vi "ChangeExecTimeCmdCluster.vi"(9 "ExecTime":string, 11 "CmdClusterIN":T2) -> (3 "CmdClusterOUT":T1)   [LabVIEW 2011]
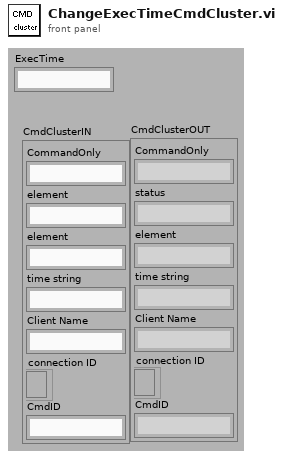
[diagram p1: front panel]
types:
  T1 = cluster{"CommandOnly":string, "status":string, "element":string, "time string":string, "Client Name":string, "connection ID":refnum<k5>, "CmdID":string}
  T2 = cluster{"CommandOnly":string, "element":string, "element":string, "time string":string, "Client Name":string, "connection ID":refnum<k5>, "CmdID":string}
  T3 = cluster{"CommandOnly":string, "element":string, "ExecTime":string, "time string":string, "Client Name":string, "connection ID":refnum<k5>, "CmdID":string}
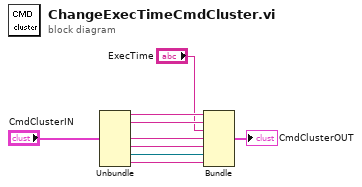
[diagram p0: block diagram]
diagram:
  n1 = Unbundle("CmdClusterIN") -> ("CommandOnly"=w8:string, "element"=w3:string, "time string"=w7:string, "Client Name"=w6:string, "connection ID"=w5:refnum<k5>, "CmdID"=w4:string)  [unwired: 1 out]
  n2 = Bundle("CommandOnly"=w8, "element"=w3, "ExecTime"="ExecTime", "time string"=w7, "Client Name"=w6, "connection ID"=w5, "CmdID"=w4) -> (→"CmdClusterOUT":T3)  [unwired: 1 out]
